vi "OpenGDSLicense_ShowAgreement.vi"(5 "error in (no error)":errorcluster) -> (16 "Accept?":bool, 19 "error out":errorcluster)   [LabVIEW 2016]
panel:
  out "ProductPicture":picture
  in  "_IDoNotAcceptAgreement":bool
  in  "_IAcceptAgreement":bool
  in  "_Cancel":bool
  in  "_Continue":bool
  out "_LicenseAgreement":string="\n20 Febrary 2014\n\nThe MIT License (MIT)\n\nCopyright (c) 2014 Open GDS Community\n\nPermission is hereby granted, free of charge, to any person obtaining a copy\n of this software and associated documentation files (the \"Software\"), to deal\n in the Software without restriction, including without limitation the rights\n to use, copy, modify, merge, publish, distribute, sublicense, and/or sell\n copies of the Software, and to permit persons to whom the Software is\n furnished to do so, subject to the following conditions:\n\nThe above copyright notice and this permission notice shall be included in\n all copies or substantial portions of the Software.\n\nTHE SOFTWARE IS PROVIDED \"AS IS\", WITHOUT WARRANTY OF ANY KIND, EXPRESS OR\n IMPLIED, INCLUDING BUT NOT LIMITED TO THE WARRANTIES OF MERCHANTABILITY,\n FITNESS FOR A PARTICULAR PURPOSE AND NONINFRINGEMENT. IN NO EVENT SHALL THE\n AUTHORS OR COPYRIGHT HOLDERS BE LIABLE FOR ANY CLAIM, DAMAGES OR OTHER\n LIABILITY, WHETHER IN AN ACTION OF CONTRACT, TORT OR OTHERWISE, ARISING FROM,\n OUT OF OR IN CONNECTION WITH THE SOFTWARE OR THE USE OR OTHER DEALINGS IN\n THE SOFTWARE.\n" caption="License Agreement"
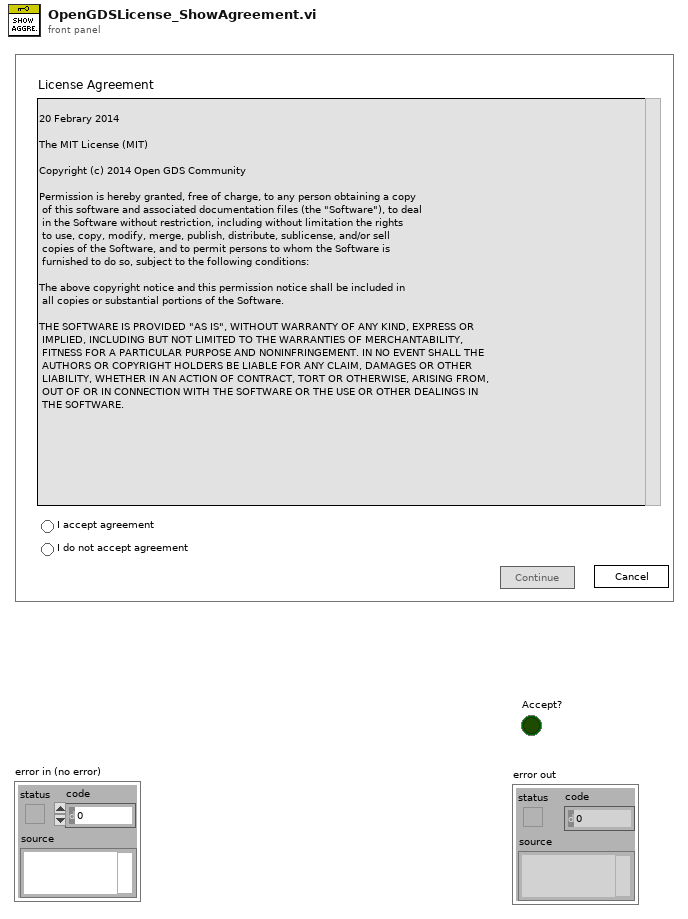
[diagram p1: front panel]
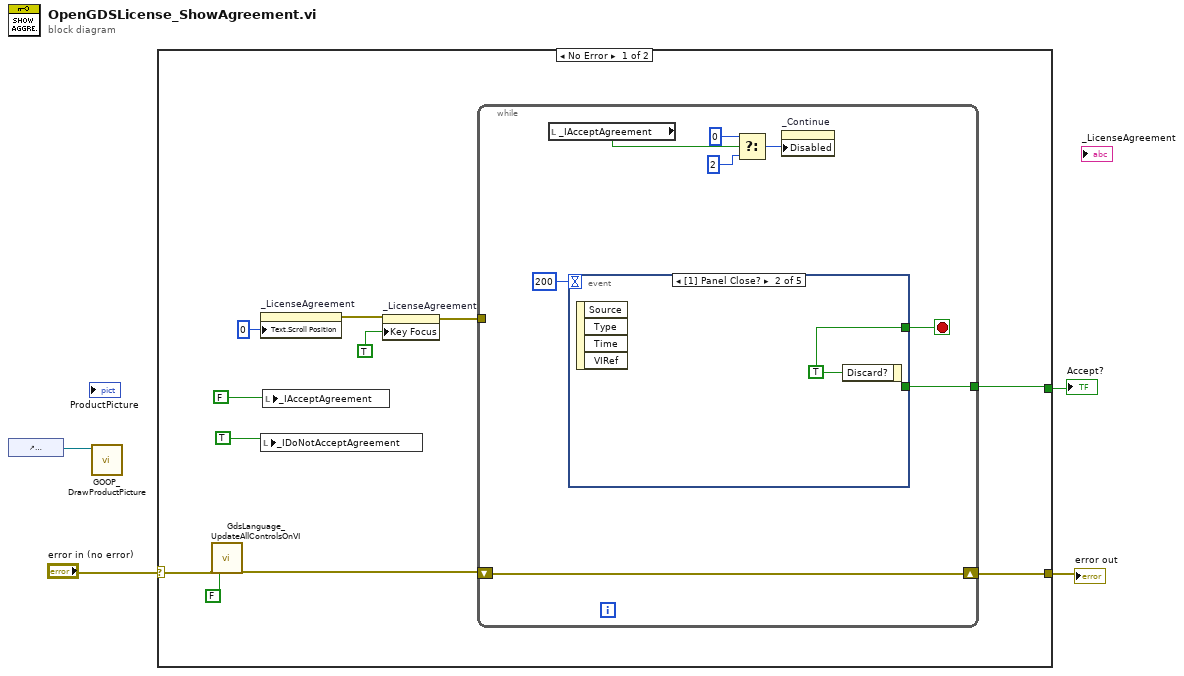
[diagram p0: block diagram]
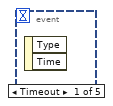
[diagram p2: hidden frame]
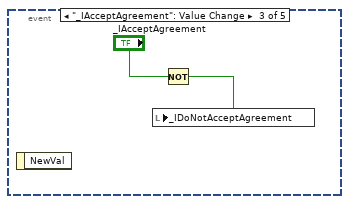
[diagram p3: hidden frame]
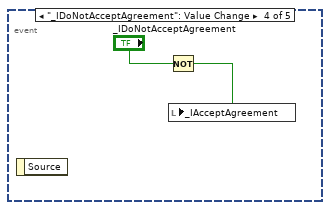
[diagram p4: hidden frame]
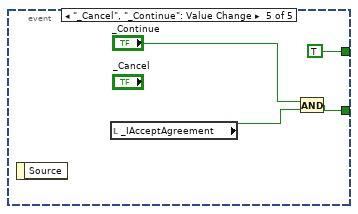
[diagram p5: hidden frame]
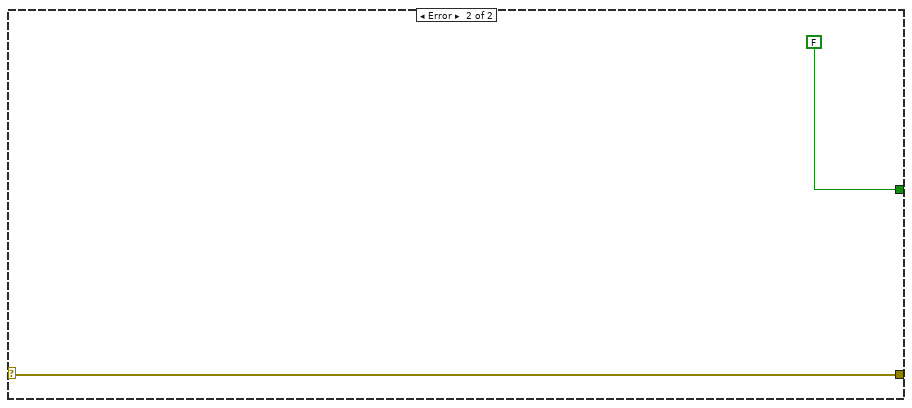
[diagram p6: hidden frame]
diagram:
  n1 = control-ref of="ProductPicture"() -> (w1:refnum<vi>)
  n2 = call <resource>:"GOOP_DrawProductPicture.vi"("ProductPictureControl"=w1) -> ()  [unwired: 10 in, 1 out]
  n3 = case shown="No Error" "error in (no error)" {
    selector: "error in (no error)" -> [w10 w34]
    tunnel: [w15 w34] -> w3
    tunnel: [w14 FALSE ("I accept agreement")] -> w2
    frame No Error {
      n4 = call <resource>:"GdsLanguage_UpdateAllControlsOnVI.vi"("error in (no error)"=w10, "CreateLanguageFile(Use this to create a languageFile)"=FALSE) -> ("error out"=w9:errorcluster)  [unwired: 16 in, 1 out]
      n5 = property on="_LicenseAgreement" class="Str"("Text.Scroll Position"=u32 0) -> (error out=w7:errorcluster)  [unwired: 2 in, 1 out]
      n6 = local write "_IDoNotAcceptAgreement"(TRUE) -> ()
      n7 = local write "_IAcceptAgreement"(FALSE) -> ()
      n8 = property on="_LicenseAgreement" class="Str"(error in=w7, "Key Focus"=TRUE) -> (error out=w5:errorcluster)  [unwired: 1 in, 1 out]
      n9 = while {
        shift-left: w9 -> [w23]
        shift-right: [w23] -> w15
        tunnel: [w20] -> w14
        tunnel: w5 -> [_]
        stop <- w21 stop-if-true
        n10 = local read "_IAcceptAgreement"() -> (w16:bool)
        n11 = event shown="[1] Panel Close?" {
          selector: _ -> [_ _ _ _ _]
          dyn-events: _ -> [_ _ _ _ _]
          timeout: 200 -> [_ _ _ _ _]
          tunnel: [_ w24 _ _ TRUE ("Discard?")] -> w21
          tunnel: [_ _ _ _ w29] -> w20
          event Timeout {
            n12 = event-data() -> ()  [unwired: 1 in, 2 out]
          }
          event Panel Close? {
            w24 = TRUE ("Discard?")
            n13 = event-data() -> ()  [unwired: 1 in, 4 out]
            n14 = event-data("Discard?"=w24) -> ()  [unwired: 1 in, 1 out]
          }
          event "_IAcceptAgreement": Value Change {
            n15 = event-data() -> ()  [unwired: 1 in, 1 out]
            n16 = Not(x="_IAcceptAgreement") -> (.not. x?=w25:bool)
            n17 = local write "_IDoNotAcceptAgreement"(w25) -> ()
          }
          event "_IDoNotAcceptAgreement": Value Change {
            n18 = event-data() -> ()  [unwired: 1 in, 1 out]
            n19 = Not(x="_IDoNotAcceptAgreement") -> (.not. x?=w28:bool)
            n20 = local write "_IAcceptAgreement"(w28) -> ()
          }
          event "_Cancel", "_Continue": Value Change {
            n21 = event-data() -> ()  [unwired: 1 in, 1 out]
            n22 = local read "_IAcceptAgreement"() -> (w31:bool)
            n23 = And(x="_Continue", y=w31) -> (x .and. y?=w29:bool)
          }
        }
        n24 = Select(t=u8 0, s=w16, f=u8 2 ("Disabled")) -> (s? t:f=w18:u8)
        n25 = property on="_Continue" class="Bool"("Disabled"=w18) -> ()  [unwired: 2 in, 2 out]
      }
    }
    frame Error {
    }
  }
  "error out" <- w3
  "Accept?" <- w2
